vi "Update UI per Reference.vi"(8 "error in (no error)":errorcluster, 11 "Analyze Results Total Counts in":refnum<class "Analyze Results Total Counts.lvclass">) -> (0 "error out":errorcluster, 3 "Analyze Results Total Counts out":refnum<class "Analyze Results Total Counts.lvclass">)   [LabVIEW 2020, in "Analyze Results Total Counts.lvclass"]
uses:
  Analyze Results Total Counts.lvclass
  Analyze Results Total Counts.lvclass/Analyze Results Total Counts.ctl
  Results Base/Analyze Results Base.lvclass
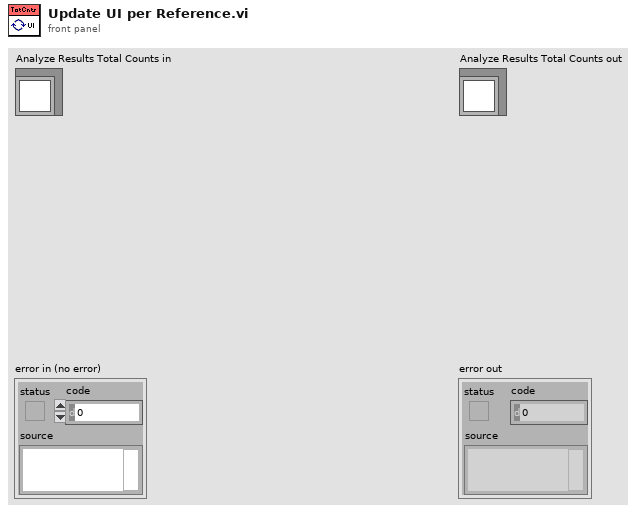
[diagram p1: front panel]
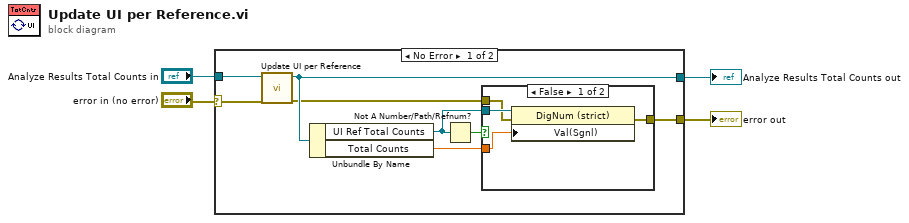
[diagram p0: block diagram]
diagram:
  n1 = case shown="No Error" "error in (no error)" {
    selector: "error in (no error)" -> [w6 w18]
    tunnel: "Analyze Results Total Counts in" -> [w12 w19]
    tunnel: [w11 w19] -> w3
    tunnel: [w7 w18] -> w2
    frame No Error {
      n2 = call-parent "Update UI per Reference.vi"("error in (no error)"=w6, "Analyze Results Base in"=w12) -> ("error out"=w8:errorcluster, "Analyze Results Base out"=w11:refnum<class "Analyze Results Total Counts.lvclass">)  [unwired: 8 in]
      n3 = Unbundle By Name(w11) -> ("UI Ref Total Counts"=w5:refnum<vi>, "Total Counts"=w9:dbl)
      n4 = Not A Number/Path/Refnum?(number/path/refnum=w5) -> (NaN/Path/Refnum?=w10:bool)
      n5 = case shown="False" w10 {
        tunnel: w5 -> [w16 _]
        tunnel: w9 -> [w15 _]
        tunnel: w8 -> [w14 w17]
        tunnel: [w13 w17] -> w7
        frame False {
          n6 = property class="DigNum (strict)"(reference=w16, error in=w14, "Val(Sgnl)"=w15) -> (error out=w13:errorcluster)  [unwired: 1 out]
        }
        frame True {
        }
      }
    }
    frame Error {
    }
  }
  "error out" <- w2
  "Analyze Results Total Counts out" <- w3
